vi "2D_array_interpolation.vi"(7 "method":i32(ring)=3 items=["nearest", "bilinear", "bicubic", "bicubic spline"], 8 "error in (no error)":errorcluster caption="错误输入（无错误）", 9 "yi":dbl, 10 "xi":dbl, 11 "2D array":dbl[][](array[numeric])) -> (0 "error out":errorcluster caption="错误输出", 1 "error":i32, 2 "f(x,y)":dbl, 4 "out-of-range":bool)   [LabVIEW 2013]
uses:
  <vilib>/gmath/interp.llb/Interpolate 2D (1d xi,yi).vi
  <vilib>/gmath/NI_Gmath.lvlib
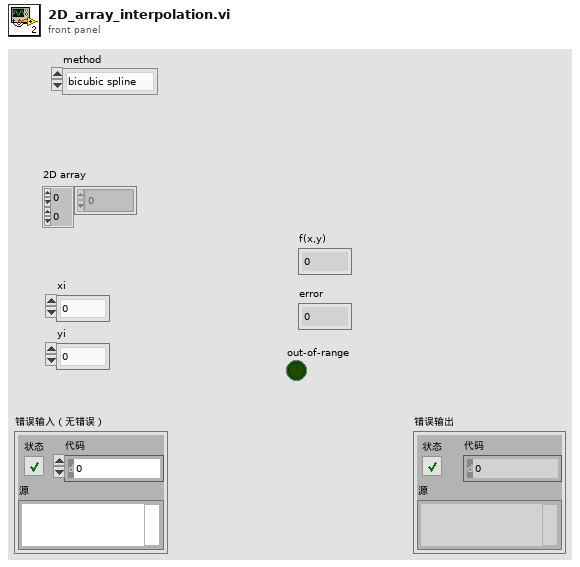
[diagram p1: front panel]
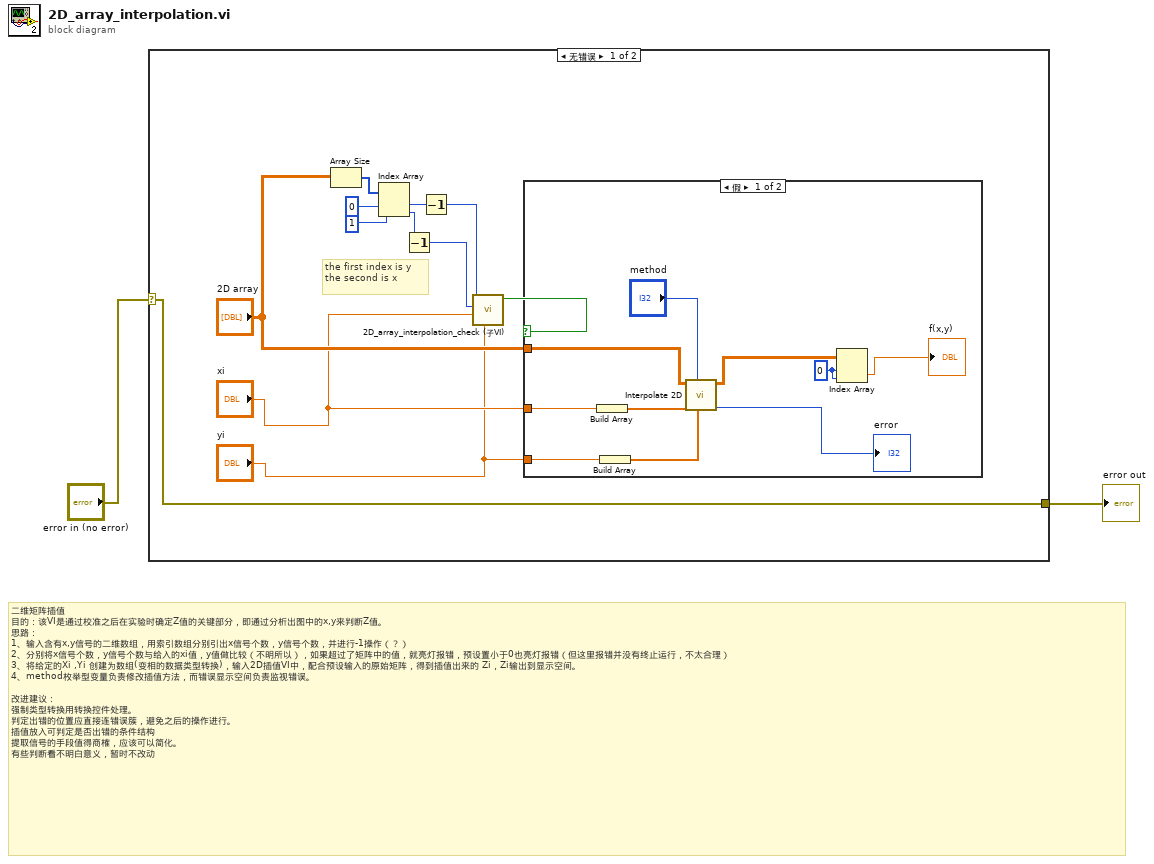
[diagram p0: block diagram]
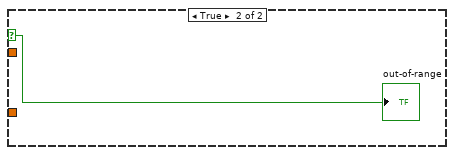
[diagram p2: hidden frame]
diagram:
  # "二维矩阵插值\n目的：该VI是通过校准之后在实验时确定Z值的关键部分，即通过分析出图中的x,y来判断Z值。\n思路：\n1、输入含有x,y信号的二维数组，用索引数组分别引出x信号个数，y信号个数，并进行-1操作（？）\n2、分别将x信号个数，y信号个数与给入的xi值，y值做比较（不明所以），如果超过了矩阵中的值，就亮灯报错，预设置小于0也亮灯报错（但这里报错并没有终止运行，不太合理）\n3、将给定的Xi ,Yi 创建为数组(变相的数据类型转换)，输入2D插值VI中，配合预设输入的原始矩阵，得到插值出来的 Zi，Zi输出到显示空间。\n4、method枚举型变量负责修改插值方法，而错误显示空间负责监视错误。\n\n改进建议：\n强制类型转换用转换控件处理。\n判定出错的位置应直接连错误簇，避免之后的操作进行。\n插值放入可判定是否出错的条件结构\n提取信号的手段值得商榷，应该可以简化。\n有些判断看不明白意义，暂时不改动"
  n1 = case shown="无错误" "error in (no error)" {
    selector: "error in (no error)" -> [w3 w26]
    tunnel: [w3 w26] -> w1
    frame No Error {
      # "the first index is y\nthe second is x"
      n2 = Array Size(array="2D array") -> (size(s)=w7:i32[])
      n3 = Index Array(array=w7, index #1=0 ("index"), index #2=1 ("index")) -> (element #1=w11:i32, element #2=w13:i32)
      n4 = Decrement(x=w13) -> (x-1=w14:i32)
      n5 = Decrement(x=w11) -> (x-1=w12:i32)
      n6 = call "2D_array_interpolation_check (子VI).vi"("yi"="yi", "xi"="xi", "x信号个数"=w14, "y信号个数"=w12) -> ("布尔"=w6:bool)  [unwired: 7 in]
      n7 = case shown="假" w6 {
        selector: w6 -> [_ w25]
        tunnel: "2D array" -> [w20 _]
        tunnel: "xi" -> [w18 _]
        tunnel: "yi" -> [w16 _]
        frame False {
          w22 = 0 ("index")
          n8 = Build Array(w18) -> (w17:dbl[])
          n9 = Build Array(w16) -> (w15:dbl[])
          n10 = call-poly <vilib>:"Interpolate 2D.vi"("yi"=w15, "method"="method", "xi"=w17, "Z"=w20) -> ("error"=→"error":i32, "zi"=w21:dbl[][])  [unwired: 3 in, 3 out]
          n11 = Index Array(array=w21, index (row)=w22, index (col)=w22) -> (element=→"f(x,y)":dbl)
        }
        frame True {
          "out-of-range" <- w25
        }
      }
    }
    frame Error {
    }
  }
  "error out" <- w1
